vi "subAcquisition_3D.vi"(5 "Z-stack cluster in":T2={"Timelapse Acquired"=1, "File path"=path "C:/Users/ZouOptics/Desktop/TEST", "Z-Stack"={"Z end"=0.0, "Step Num"=1, "Step Size"=2.0, "Z0"=3471.0, "z-stack?"=FALSE}, "Frames to avg."=20, "Image Info Ref"=refnum, "Camera Ctrl"={"Chosen Camera"=0, "ROI selection"=0, "Live"=FALSE, "ROI define"=FALSE, "Snap"=FALSE, "ROI update"=FALSE, "ROI previous "=FALSE, "ROI"={"Bin"=2, "ROI"={"x offset"=256, "y offset"=256, "x width"=512, "y width"=512}}, "Exposure (ms)"=100.0, "Symmetrical"=FALSE, "Autoscale"=TRUE, "Scale"={"Scale.Min"=0, "Scale.Max"=6038}}} {"Camera Ctrl"."Scale"."Scale.Max" min=1 max=5000 step=1; "Camera Ctrl"."Scale"."Scale.Min" min=1 max=5000 step=1; "Camera Ctrl"."Exposure (ms)" min=1.0 max=5000.0 step=1.0; "Camera Ctrl"."ROI"."ROI"."x offset" min=1 max=512 step=1; "Camera Ctrl"."ROI"."ROI"."y offset" min=1 max=512 step=1; "Camera Ctrl"."ROI"."ROI"."x width" min=1 max=512 step=1; "Camera Ctrl"."ROI"."ROI"."y width" min=1 max=512 step=1; "Camera Ctrl"."ROI"."Bin" items=["1x1"=1, "2x2"=2, "4x4"=4]; "Camera Ctrl"."ROI selection" items=["Full ROI", "Central quad", "Confocal"]; "Camera Ctrl"."Chosen Camera" items=["Left", "Right"]}, 6 "Ti-E cluster":T3, 7 "Stage cluster":T1={"XY tiling"={"Tiling?"=FALSE, "YY/XX"=[1, 1], "X0Y0"=[-1.0, -12.0, 0.0]}, "Stage Status Ref"=refnum}, 8 "error in":errorcluster, 10 "Z Stack Aquired Refnum":refnum<vi>, 11 "Handle in":u32) -> (0 "error out":errorcluster)   [LabVIEW 2015]
panel:
  # "X"
  # "Y"
  # "X"
  # "Y"
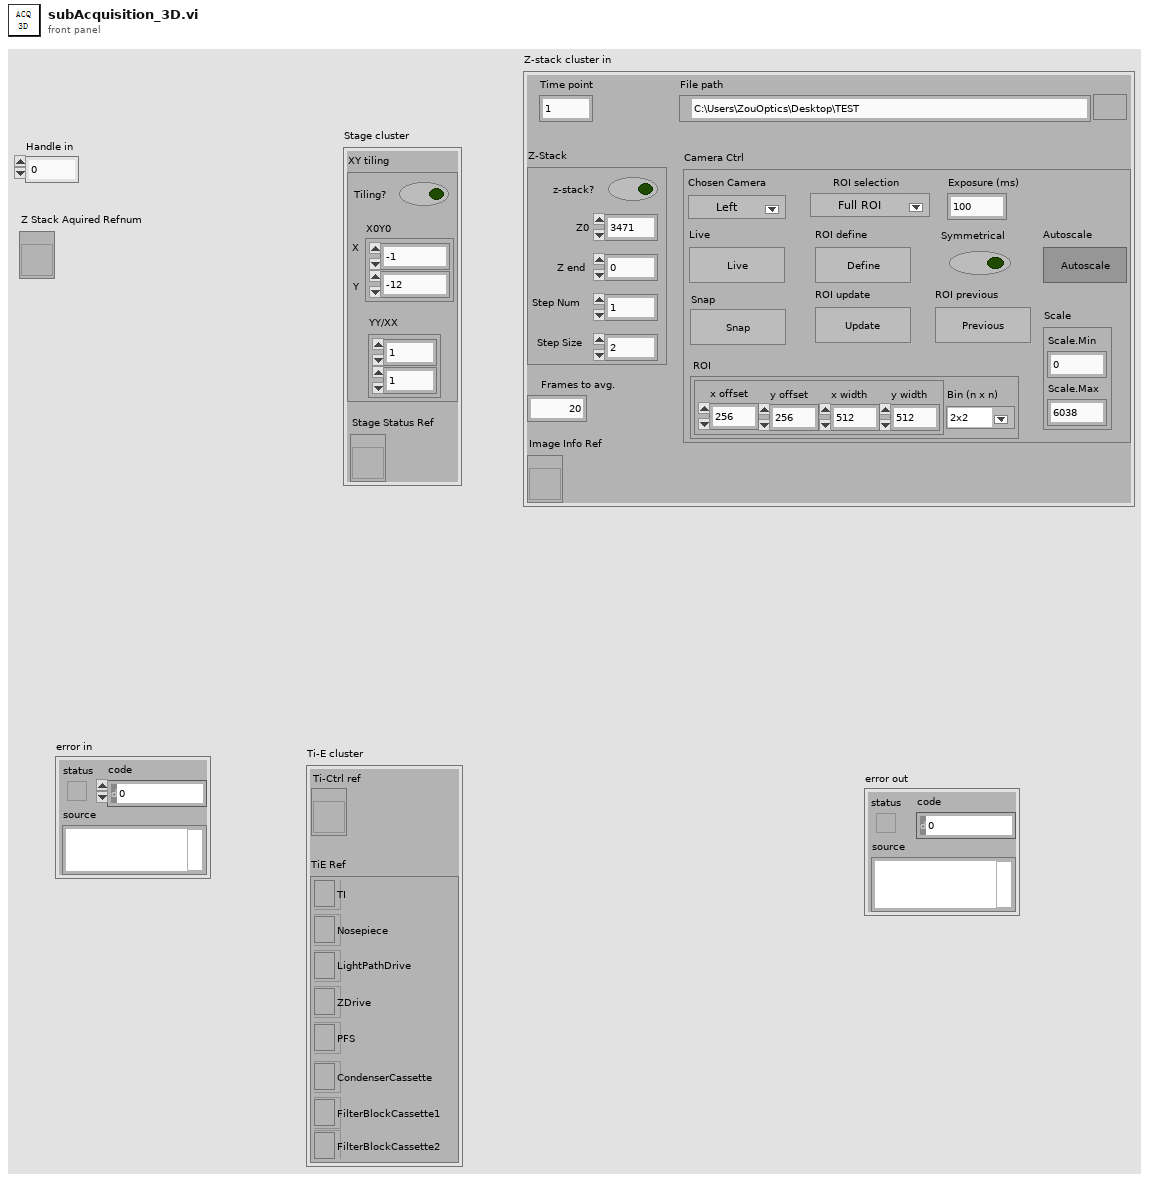
[diagram p1: front panel]
types:
  T1 = cluster{"XY tiling":cluster{"Tiling?":bool, "YY/XX":i32[], "X0Y0":dbl[]}, "Stage Status Ref":refnum<vi>}
  T2 = cluster{"Timelapse Acquired":i32, "File path":path, "Z-Stack":cluster{"Z end":dbl, "Step Num":i32, "Step Size":dbl, "Z0":dbl, "z-stack?":bool}, "Frames to avg.":i32, "Image Info Ref":refnum<vi>, "Camera Ctrl":cluster{"Chosen Camera":u32, "ROI selection":u16, "Live":bool, "ROI define":bool, "Snap":bool, "ROI update":bool, "ROI previous ":bool, "ROI":cluster{"Bin":u16, "ROI":cluster{"x offset":i32, "y offset":i32, "x width":i32, "y width":i32}}, "Exposure (ms)":dbl, "Symmetrical":bool, "Autoscale":bool, "Scale":cluster{"Scale.Min":i32, "Scale.Max":i32}}}
  T3 = cluster{"Ti-Ctrl ref":refnum<vi>, "TiE Ref":cluster{"TI":refnum<k7>, "Nosepiece":refnum<k7>, "LightPathDrive":refnum<k7>, "ZDrive":refnum<k7>, "PFS":refnum<k7>, "CondenserCassette":refnum<k7>, "FilterBlockCassette1":refnum<k7>, "FilterBlockCassette2":refnum<k7>}}
  T4 = cluster{"Obj":u16, "Cube Bottom":u16, "Cube Top":u16, "PFS-Ctrl":cluster{"PFS IO":bool, "PSF Err":bool, "PSF Pos":u32}, "Z-Ctrl":cluster{"Z-pos":dbl, "Home":bool, "Sensitivity":u8}, "Condenser":u16, "Lightpath":enum32{"EYE", "L100", "R100", "L80"}}
  T5 = cluster{"Bin":u16, "ROI":cluster{"x offset":i32, "y offset":i32, "x width":i32, "y width":i32}}
  T6 = cluster{"Tiling?":bool, "YY/XX":i32[], "X0Y0":dbl[]}
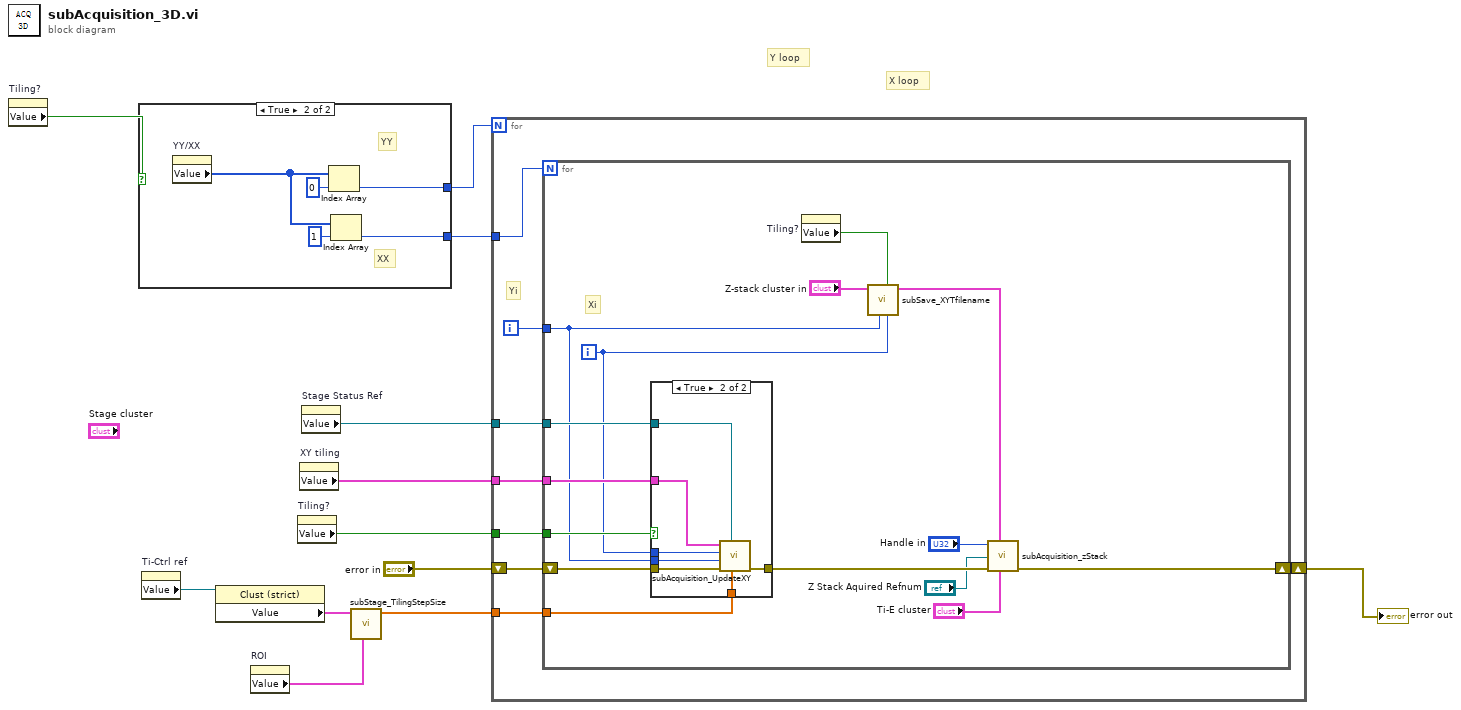
[diagram p0: block diagram]
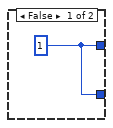
[diagram p2: hidden frame]
diagram:
  # "X loop"
  # "Y loop"
  n1 = property on="Tiling?" class="Bool (strict)"() -> ("Value"=w4:bool)  [unwired: 2 in, 2 out]
  n2 = case shown="True" w4 {
    tunnel: [w13 w17] -> w12
    tunnel: [w13 w15] -> w11
    frame False {
      w13 = 1 ("XX")
    }
    frame True {
      # "XX"
      # "YY"
      n3 = property on="YY/XX" class="Arr (strict)"() -> ("Value"=w14:i32[])  [unwired: 2 in, 2 out]
      n4 = Index Array(array=w14, index=0) -> (element=w17:i32)
      n5 = Index Array(array=w14, index=1) -> (element=w15:i32)
    }
  }
  n6 = property on="Ti-Ctrl ref" class="LVObjRef (strict)"() -> ("Value"=w6:refnum<vi>)  [unwired: 2 in, 2 out]
  n7 = property class="Clust (strict)"(reference=w6) -> ("Value"=w8:T4)  [unwired: 1 in, 2 out]
  n8 = property on="ROI" class="Clust (strict)"() -> ("Value"=w5:T5)  [unwired: 2 in, 2 out]
  n9 = property on="Tiling?" class="Bool (strict)"() -> ("Value"=w3:bool)  [unwired: 2 in, 2 out]
  n10 = property on="XY tiling" class="Clust (strict)"() -> ("Value"=w2:T6)  [unwired: 2 in, 2 out]
  n11 = property on="Stage Status Ref" class="LVObjRef (strict)"() -> ("Value"=w1:refnum<vi>)  [unwired: 2 in, 2 out]
  n12 = call "subStage_TilingStepSize.vi"("ROI"=w5, "TI-Ctrl"=w8) -> ("Tiling step size (mm)"=w7:dbl[])  [unwired: 9 in]
  n13 = for {
    N: w12 -> [_]
    shift-right: [w25] -> w9
    shift-left: "error in" -> [w26]
    tunnel: w11 -> [w24]
    tunnel: w2 -> [w22]
    tunnel: w7 -> [w21]
    tunnel: w3 -> [w20]
    tunnel: w1 -> [w19]
    i -> [w23]
    # "Yi"
    n14 = for {
      N: w24 -> [_]
      tunnel: w23 -> [w29]
      shift-right: [w39] -> w25
      shift-left: w26 -> [w41]
      tunnel: w22 -> [w40]
      tunnel: w21 -> [w37]
      tunnel: w20 -> [w36]
      tunnel: w19 -> [w34]
      i -> [w28]
      # "Xi"
      n15 = case shown="True" w36 {
        tunnel: w41 -> [w42 w49]
        tunnel: w40 -> [_ w44]
        tunnel: [w42 w48] -> w38
        tunnel: w37 -> [_ w47]
        tunnel: w28 -> [_ w46]
        tunnel: w29 -> [_ w45]
        tunnel: w34 -> [_ w43]
        frame False {
        }
        frame True {
          n16 = call "subAcquisition_UpdateXY.vi"("Grid step size (mm)"=w47, "Stage Status Ref"=w43, "error in"=w49, "Yj"=w45, "Xi"=w46, "XY tiling"=w44) -> ("error out"=w48:errorcluster)  [unwired: 5 in]
        }
      }
      n17 = property on="Tiling?" class="Bool (strict)"() -> ("Value"=w32:bool)  [unwired: 2 in, 2 out]
      n18 = call "subSave_XYTfilename.vi"("Xi"=w28, "Tiling?"=w32, "Yi"=w29, "Z-stack cluster in"="Z-stack cluster in") -> ("Z-stack cluster out"=w31:T2)  [unwired: 7 in]
      n19 = call "subAcquisition_zStack.vi"("Ti-E cluster"="Ti-E cluster", "Z-stack cluster"=w31, "error in"=w38, "Z Stack Aquired Refnum"="Z Stack Aquired Refnum", "Handle in"="Handle in") -> ("error out"=w39:errorcluster)  [unwired: 6 in]
    }
  }
  "error out" <- w9
